vi "EndTrack.vi"(8 "error in (no error)":errorcluster, 10 "EndingCameraFrame":i32, 11 "StimulusObject in":refnum<class "StimulusObject.lvclass">) -> (0 "error out":errorcluster, 3 "StimulusObject out":refnum<class "StimulusObject.lvclass">)   [LabVIEW 2019, in "StimulusObject.lvclass"]
uses:
  StimulusObject.lvclass
  StimulusObject.lvclass/StimulusObject.ctl
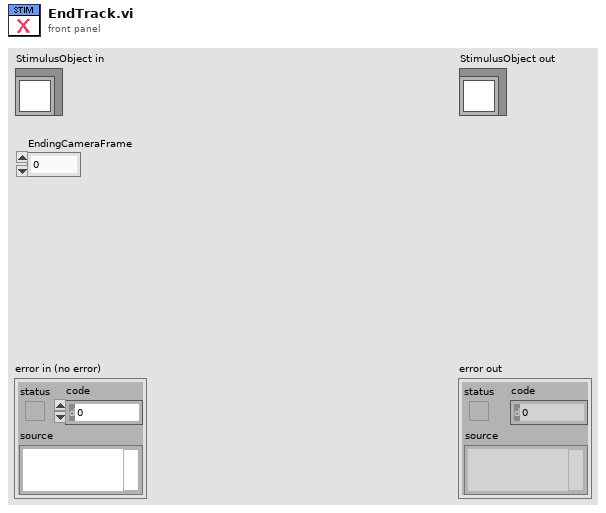
[diagram p1: front panel]
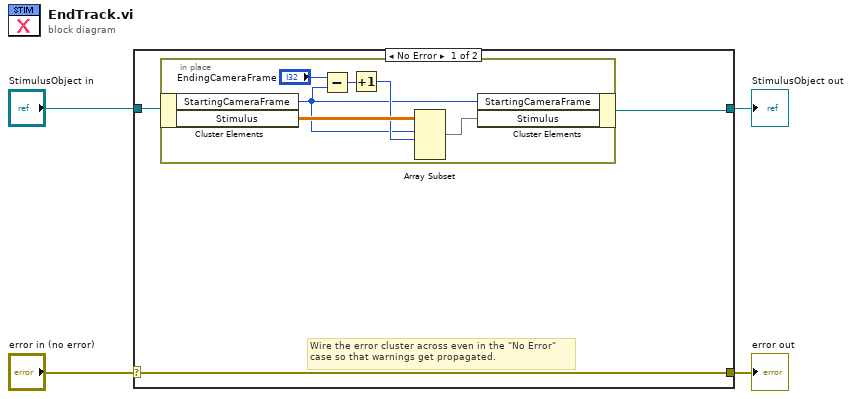
[diagram p0: block diagram]
diagram:
  n1 = case shown="No Error" "error in (no error)" {
    selector: "error in (no error)" -> [w7 w15]
    tunnel: [w7 w15] -> w3
    tunnel: [w5 w14] -> w1
    tunnel: "StimulusObject in" -> [w6 w14]
    frame No Error {
      # "Wire the error cluster across even in the \"No Error\"\ncase so that warnings get propagated."
      n2 = in-place {
        n3 = in-place-cluster #1(w6) -> ("StartingCameraFrame"=w8:i32, "Stimulus"=w12:sgl[][])
        n4 = Subtract(x="EndingCameraFrame", y=w8) -> (x-y=w11:i32)
        n5 = Increment(x=w11) -> (x+1=w10:i32)
        n6 = Array Subset(array=w12, index (row)=w8, length (row)=w10) -> (w9:sgl[][])  [unwired: 2 in]
        n7 = in-place-cluster #1("StartingCameraFrame"=w8, "Stimulus"=w9) -> (w5:refnum<class "StimulusObject.lvclass">)
      }
    }
    frame Error {
    }
  }
  "error out" <- w3
  "StimulusObject out" <- w1
